vi "Configure User Defined Waveform.vi"(0 "VISA resource name":refnum<visa-resource-name>, 5 "Create/Delete Waveform (0:Create)":u16(ring) items=["Create", "Delete", "Delete All"], 7 "Waveform Name (\"ARB1\")":string="ARB1", 9 "Waveform Data":dbl[](array[numeric]), 11 "error in (no error)":errorcluster) -> (4 "VISA resource name out":refnum<visa-resource-name>, 15 "error out":errorcluster)   [LabVIEW 2013, in "California Instruments iX Series.lvlib"]
doc: "Creates or delete user defined waveform."
uses:
  <instrlib>/California Instruments iX Series/California Instruments iX Series.lvlib
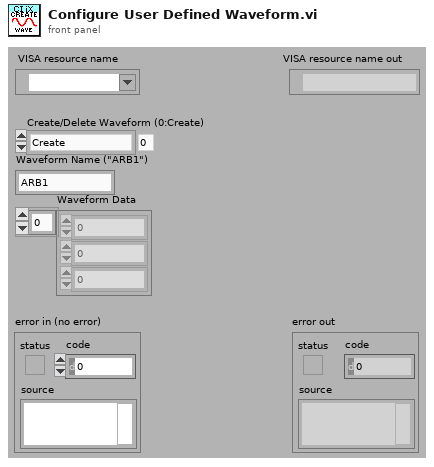
[diagram p1: front panel]
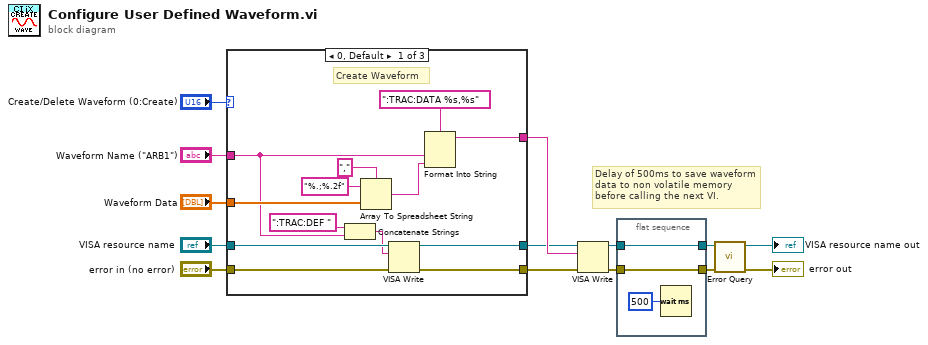
[diagram p0: block diagram]
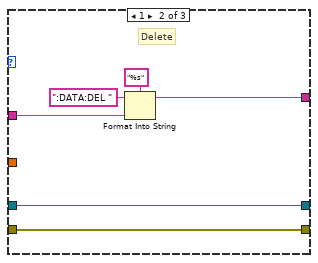
[diagram p2: hidden frame]
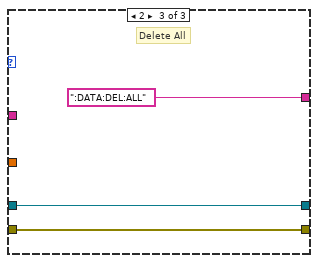
[diagram p3: hidden frame]
diagram:
  # "Delay of 500ms to save waveform data to non volatile memory before calling the next VI."
  n1 = case shown="0, Default" "Create/Delete Waveform (0:Create)" {
    tunnel: "Waveform Name (\"ARB1\")" -> [w17 w32 _]
    tunnel: "Waveform Data" -> [w26 _ _]
    tunnel: [w22 w30 ":DATA:DEL:ALL"] -> w10
    tunnel: [w21 w29 w35] -> w5
    tunnel: [w20 w28 w34] -> w4
    tunnel: "VISA resource name" -> [w19 w29 w35]
    tunnel: "error in (no error)" -> [w18 w28 w34]
    frame 0, Default {
      # "Create Waveform"
      n2 = Concatenate Strings(":TRAC:DEF " ("string"), w17) -> (w15:string)
      n3 = Array To Spreadsheet String(delimiter (Tab)=",", array=w26, 3:"%.;%.2f" ("format string")) -> (spreadsheet string=w23:string)
      n4 = VISA Write(VISA resource name=w19, write buffer=w15, error in (no error)=w18) -> (VISA resource name out=w21:refnum<visa-resource-name>, error out=w20:errorcluster)  [unwired: 1 out]
      n5 = Format Into String(format string=":TRAC:DATA %s,%s", w17, w23) -> (resulting string=w22:string)  [unwired: 2 in, 1 out]
    }
    frame 1 {
      # "Delete"
      n6 = Format Into String(format string="%s", initial string=":DATA:DEL ", w32) -> (resulting string=w30:string)  [unwired: 1 in, 1 out]
    }
    frame 2 {
      # "Delete All"
    }
  }
  n7 = VISA Write(VISA resource name=w5, write buffer=w10, error in (no error)=w4) -> (VISA resource name out=w9:refnum<visa-resource-name>, error out=w7:errorcluster)  [unwired: 1 out]
  n8 = flat-sequence {
    tunnel: w9 -> [w39]
    tunnel: [w39] -> w8
    tunnel: w7 -> [w38]
    tunnel: [w38] -> w6
    frame #0 {
      n9 = Wait (ms)(milliseconds to wait=u32 500) -> ()  [unwired: 1 out]
    }
  }
  n10 = call <instrlib>:"Error Query.vi"("error in (no error)"=w6, "VISA resource name"=w8) -> ("error out"=→"error out":errorcluster, "VISA resource name out"=→"VISA resource name out":refnum<visa-resource-name>)  [unwired: 6 in, 2 out]
